vi "GraphSetting Conv AutoScale.vi"(11 "XScale.ScaleFit":u8) -> (3 "自動スケール?":bool)   [LabVIEW 2014]
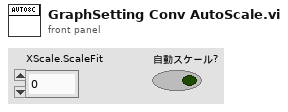
[diagram p1: front panel]
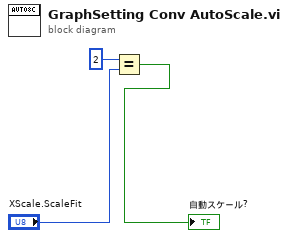
[diagram p0: block diagram]
diagram:
  n1 = Equal?(x=u8 2, y="XScale.ScaleFit") -> (x = y?=→"自動スケール?":bool)
